vi "Configure Average.vi"(7 "Average On":bool, 8 "error in (no error)":errorcluster, 10 "Number of Averages":i32, 11 "VNA-Ag87xx in":refnum<class "VNA-Ag87xx.lvclass">) -> (0 "error out":errorcluster, 3 "VNA-Ag87xx out":refnum<class "VNA-Ag87xx.lvclass">)   [LabVIEW 2020, in "VNA-Ag87xx.lvclass"]
doc: "Configures the average to use for the sweep"
uses:
  VNA-Ag87xx.lvclass
  C:/Sandbox/RF Bench/Source Code/WiSpry Test Framework/Instruments/Instrument.lvclass
  C:/Sandbox/RF Bench/Source Code/WiSpry Test Framework/Instruments/Vector Network Analyzer/Vector Network Analyzer.lvclass
  Instrument.lvclass/Instrument.ctl
  Vector Network Analyzer.lvclass/Vector Network Analyzer.ctl
  Instrument.lvclass
  Vector Network Analyzer.lvclass
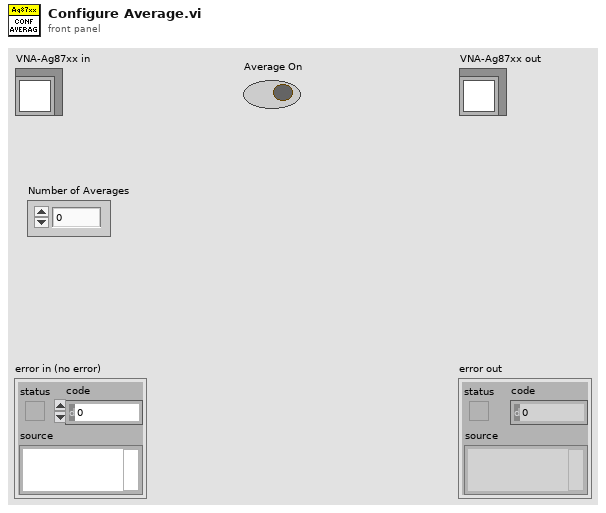
[diagram p1: front panel]
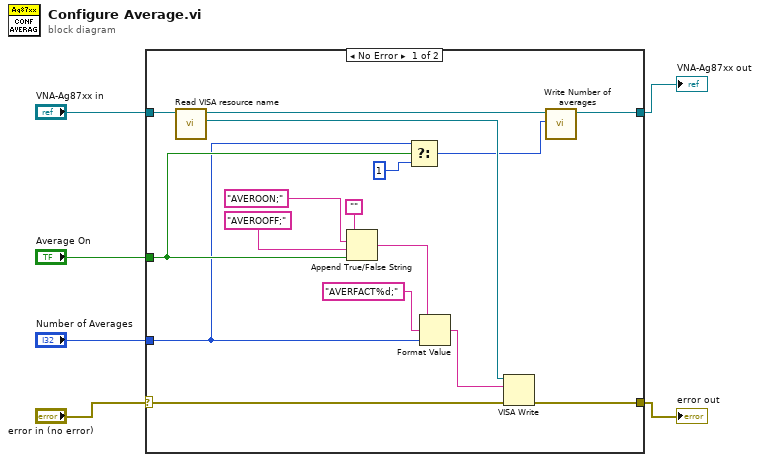
[diagram p0: block diagram]
diagram:
  n1 = case shown="No Error" "error in (no error)" {
    selector: "error in (no error)" -> [w16 w23]
    tunnel: [w7 w24] -> w4
    tunnel: "VNA-Ag87xx in" -> [w22 w24]
    tunnel: [w17 w23] -> w5
    tunnel: "Number of Averages" -> [w11 _]
    tunnel: "Average On" -> [w12 _]
    frame No Error {
      n2 = call "Read VISA resource name.vi"("Instrument in"=w22) -> ("VISA resource name"=w15:refnum<visa-resource-name>, "Instrument out"=w8:refnum<class "VNA-Ag87xx.lvclass">)  [unwired: 9 in]
      n3 = Append True/False String(1:w12, 2:"AVEROOFF;", 3:"AVEROON;", 4:"") -> (0:w13:string)
      n4 = Select(t=w11, s=w12, f=1) -> (s? t:f=w9:i32)
      n5 = Format Value(string ("")=w13, format string="AVERFACT%d;", value (0)=w11) -> (output string=w14:string)
      n6 = VISA Write(VISA resource name=w15, write buffer=w14, error in (no error)=w16) -> (error out=w17:errorcluster)  [unwired: 2 out]
      n7 = call "Write Number of averages.vi"("Number of averages"=w9, "Vector Network Analyzer in"=w8) -> ("Vector Network Analyzer out"=w7:refnum<class "VNA-Ag87xx.lvclass">)  [unwired: 9 in]
    }
    frame Error {
    }
  }
  "error out" <- w5
  "VNA-Ag87xx out" <- w4
